vi "Read Current.vi"(10 "task in":refnum<k21>, 11 "physical channels":tag="Dev2/ai0") -> (2 "task out":refnum<k21>, 3 "data":dbl[](array[numeric]) format="%0.2f")   [LabVIEW 2018]
uses:
  <vilib>/DAQmx/read.llb/DAQmx Read (Analog 1D DBL NChan 1Samp).vi
  <vilib>/DAQmx/create/channels.llb/DAQmx Create Channel (AI-Current-Basic).vi
  <vilib>/DAQmx/miscellaneous.llb/DAQmx Fill In Error Info.vi
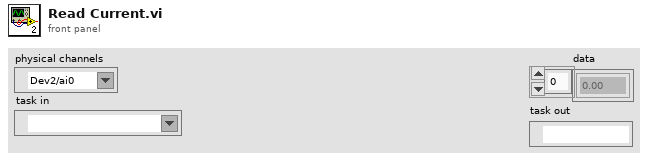
[diagram p1: front panel]
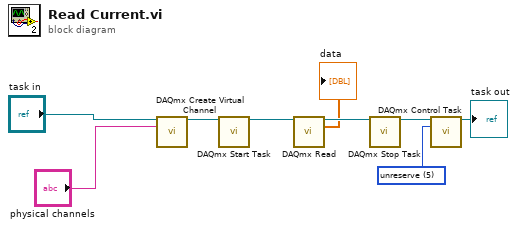
[diagram p0: block diagram]
diagram:
  w4 = 5 items=["verify"=2, "reserve"=4, "commit"=3, "unreserve"=5, "abort"=6] ("action")
  n1 = call-poly <vilib>:"DAQmx Create Virtual Channel.vi"("task in"="task in", "physical channels"="physical channels") -> ("task out"=w8:refnum<k21>)  [unwired: 12 in, 1 out]
  n2 = call <vilib>:"DAQmx Start Task.vi"("task/channels in"=w8) -> ("task out"=w9:refnum<k21>)  [unwired: 13 in, 1 out]
  n3 = call-poly <vilib>:"DAQmx Read.vi"("task/channels in"=w9) -> ("task out"=w7:refnum<k21>, "data"=→"data":dbl[])  [unwired: 12 in, 1 out]
  n4 = call <vilib>:"DAQmx Stop Task.vi"("task/channels in"=w7) -> ("task out"=w3:refnum<k21>)  [unwired: 13 in, 1 out]
  n5 = call <vilib>:"DAQmx Control Task.vi"("task/channels in"=w3, "action"=w4) -> ("task out"=→"task out":refnum<k21>)  [unwired: 12 in, 1 out]
